vi "AddTreeItem.vi"(4 "Item Indent":i32=1, 5 "Path":path, 7 "error in":errorcluster, 8 "Path to start the search":path, 9 "Parent Tag":string, 10 "Tree In":refnum<vi>) -> (0 "error out":errorcluster, 2 "Folders Found":path[](array[path]), 3 "Tree Out":refnum<vi>)   [LabVIEW 2010]
doc: "This VI populates the tree control with the folders and their respective subfolders and files. \nIf Pattern to search control has a valid file type extension, only those files will be displayed."
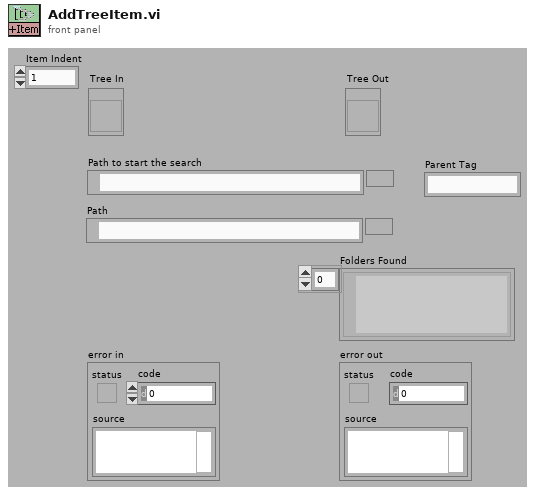
[diagram p1: front panel]
types:
  T1 = cluster{"Left Cell String":string, "Child Text":string[], "Child Tag":string, "Item Indent":i32, "Child Only?":bool, "Glyph Index":i32}
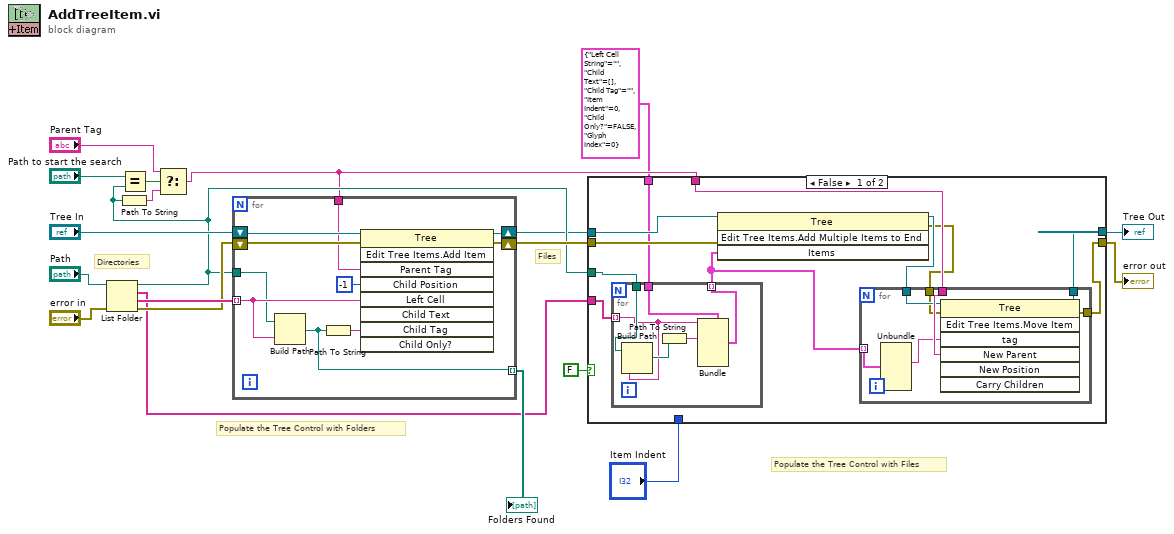
[diagram p0: block diagram]
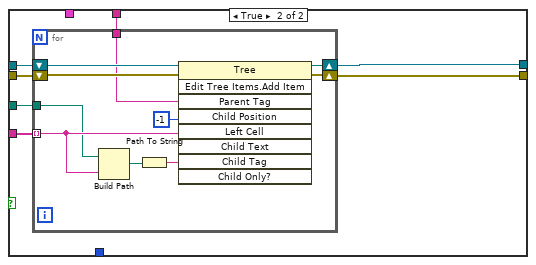
[diagram p2: hidden frame]
diagram:
  # "Populate the Tree Control with Files"
  # "Populate the Tree Control with Folders"
  # "Files"
  # "Directories"
  n1 = List Folder(path="Path", error in="error in") -> (path out=w7:path, filenames=w12:string[], folder names=w18:string[], error out=w15:errorcluster)  [unwired: 2 in]
  n2 = Path To String(path=w7) -> (string=w8:string)
  n3 = Equal?(x="Path to start the search", y=w7) -> (x = y?=w9:bool)
  n4 = Select(t="Parent Tag", s=w9, f=w8) -> (s? t:f=w6:string)
  n5 = for {
    tunnel: w7 -> [w26]
    tunnel: [w28] -> w20 mode=indexing
    tunnel: w18 -> [w29] mode=indexing
    tunnel: w6 -> [w21]
    shift-right: [w24] -> w13
    shift-left: w15 -> [w23]
    shift-right: [w22] -> w2
    shift-left: "Tree In" -> [w25]
    n6 = Build Path(base path=w26, name or relative path=w29) -> (appended path=w28:path)
    n7 = Path To String(path=w28) -> (string=w27:string)
    n8 = invoke on="Invoke Node" class="Tree" method="Edit Tree Items.Add Item"(reference=w25, error in=w23, "Parent Tag"=w21, "Child Position"=-1 ("Child Posn"), "Left Cell"=w29, "Child Tag"=w27) -> (reference out=w22:refnum<vi>, error out=w24:errorcluster)  [unwired: 3 in, 7 out]
  }
  "Folders Found" <- w20
  n9 = case shown="False" FALSE {
    tunnel: [w31 w61] -> w17
    tunnel: w2 -> [w41 w60]
    tunnel: [w34 w59] -> w3
    tunnel: w13 -> [w40 w58]
    tunnel: w12 -> [w38 w57]
    tunnel: w7 -> [w37 w56]
    tunnel: w6 -> [w36 w55]
    tunnel: T1 {"Left Cell String"="", "Child Text"=[], "Child Tag"="", "Item Indent"=0, "Child Only?"=FALSE, "Glyph Index"=0} ("Item") -> [w39 _]
    tunnel: "Item Indent" -> [_ _]
    frame False {
      n10 = for {
        tunnel: w39 -> [w54]
        tunnel: w38 -> [w51] mode=indexing
        tunnel: w37 -> [w52]
        tunnel: [w50] -> w33 mode=indexing
        n11 = Build Path(base path=w52, name or relative path=w51) -> (appended path=w53:path)
        n12 = Path To String(path=w53) -> (string=w49:string)
        n13 = Bundle(cluster=w54, "Left Cell String"=w51, "Child Tag"=w49) -> (w50:T1)  [unwired: 4 in]
      }
      n14 = invoke on="Invoke Node" class="Tree" method="Edit Tree Items.Add Multiple Items to End"(reference=w41, error in=w40, "Items"=w33) -> (reference out=w35:refnum<vi>, error out=w32:errorcluster)  [unwired: 1 in, 2 out]
      n15 = for {
        tunnel: w36 -> [w48]
        tunnel: w35 -> [w47]
        tunnel: [w46] -> w34
        tunnel: w33 -> [w45] mode=indexing
        tunnel: w32 -> [w43]
        tunnel: [w42] -> w31
        n16 = Unbundle(w45) -> ("Child Tag"=w44:string)  [unwired: 5 out]
        n17 = invoke on="Invoke Node" class="Tree" method="Edit Tree Items.Move Item"(reference=w47, error in=w43, "tag"=w44, "New Parent"=w48) -> (reference out=w46:refnum<vi>, error out=w42:errorcluster)  [unwired: 3 in, 5 out]
      }
    }
    frame True {
      n18 = for {
        tunnel: w57 -> [w66] mode=indexing
        tunnel: w56 -> [w65]
        shift-right: [w70] -> w61
        shift-left: w58 -> [w71]
        shift-right: [w63] -> w59
        shift-left: w60 -> [w64]
        tunnel: w55 -> [w62]
        n19 = Build Path(base path=w65, name or relative path=w66) -> (appended path=w68:path)
        n20 = Path To String(path=w68) -> (string=w67:string)
        n21 = invoke on="Invoke Node" class="Tree" method="Edit Tree Items.Add Item"(reference=w64, error in=w71, "Parent Tag"=w62, "Child Position"=-1 ("Child Posn"), "Left Cell"=w66, "Child Tag"=w67) -> (reference out=w63:refnum<vi>, error out=w70:errorcluster)  [unwired: 3 in, 7 out]
      }
    }
  }
  "error out" <- w17
  "Tree Out" <- w3
